vi "TimeDate.vi"() -> (2 "time_Y/M/D S":string, 3 "time_YMD":string)   [LabVIEW 2018]
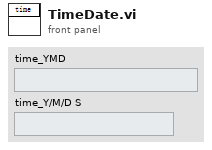
[diagram p1: front panel]
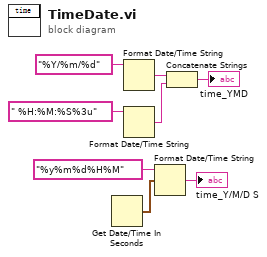
[diagram p0: block diagram]
diagram:
  n1 = Get Date/Time In Seconds() -> (seconds since 1Jan1904=w3:timestamp)
  n2 = Format Date/Time String(time format string (%c)="%Y/%m/%d" ("时间格式字符串(%c)")) -> (date/time string=w7:string)  [unwired: 2 in]
  n3 = Format Date/Time String(time format string (%c)=" %H:%M:%S%3u" ("时间格式字符串(%c)")) -> (date/time string=w6:string)  [unwired: 2 in]
  n4 = Format Date/Time String(time format string (%c)="%y%m%d%H%M" ("时间格式字符串(%c)"), seconds (now)=w3) -> (date/time string=→"time_Y/M/D S":string)  [unwired: 1 in]
  n5 = Concatenate Strings(w7, w6) -> (→"time_YMD":string)
